vi "DriveNetwork.vi"(8 "error in (no error)":errorcluster) -> (0 "error out":errorcluster)   [LabVIEW 2023]
doc: "Network for Drive\n\nInputs:\n -- Error in -- Error cluster -- propagated error input\n\nOutputs:\n -- Error out -- Error cluster -- progated error output"
uses:
  DriveGlobal.vi
  <vilib>/Rock Robotics/Network Tables/NT Get Topic.vi
  <vilib>/Rock Robotics/Network Tables/NT Get PublishHandle.vi
  <vilib>/Rock Robotics/Network Tables/NT_LL_Write Number.vi
  <vilib>/Rock Robotics/Network Tables/NT Check Errors.vi
  <vilib>/Rock Robotics/WPI/ThirdParty/JAS_Junk/TrajLib/Trajectory_Library.lvlib
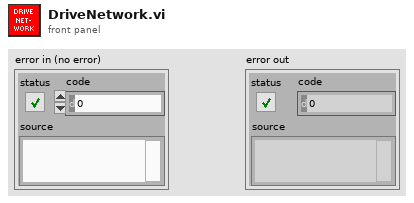
[diagram p1: front panel]
types:
  T1 = typedef "Trajectory_Library.lvlib/SWERVE_DRIVE_KINEMATICS.ctl" = cluster{"NumModules":i32, "InverseKinematics":T2, "ForwardKinematics":T2, "Modules":T3[], "PrevCoR":T3, "SavedModuleStates":T4[]}
  T2 = typedef "NI_Matrix.lvlib/RealMatrix.ctl" = dbl[][]
  T3 = typedef "Trajectory_Library.lvlib/TRANSLATION2D.ctl" = cluster{"X":dbl, "Y":dbl}
  T4 = typedef "Trajectory_Library.lvlib/SWERVE_DRIVE_MODULE_STATE.ctl" = cluster{"Speed":dbl, "Angle":T5}
  T5 = typedef "Trajectory_Library.lvlib/ROTATION2D.ctl" = cluster{"VALUE":dbl, "COS":dbl, "SIN":dbl}
  T6 = typedef "Trajectory_Library.lvlib/CHASSIS_SPEEDS.ctl" = cluster{"vX":dbl, "vY":dbl, "vOmega":dbl}
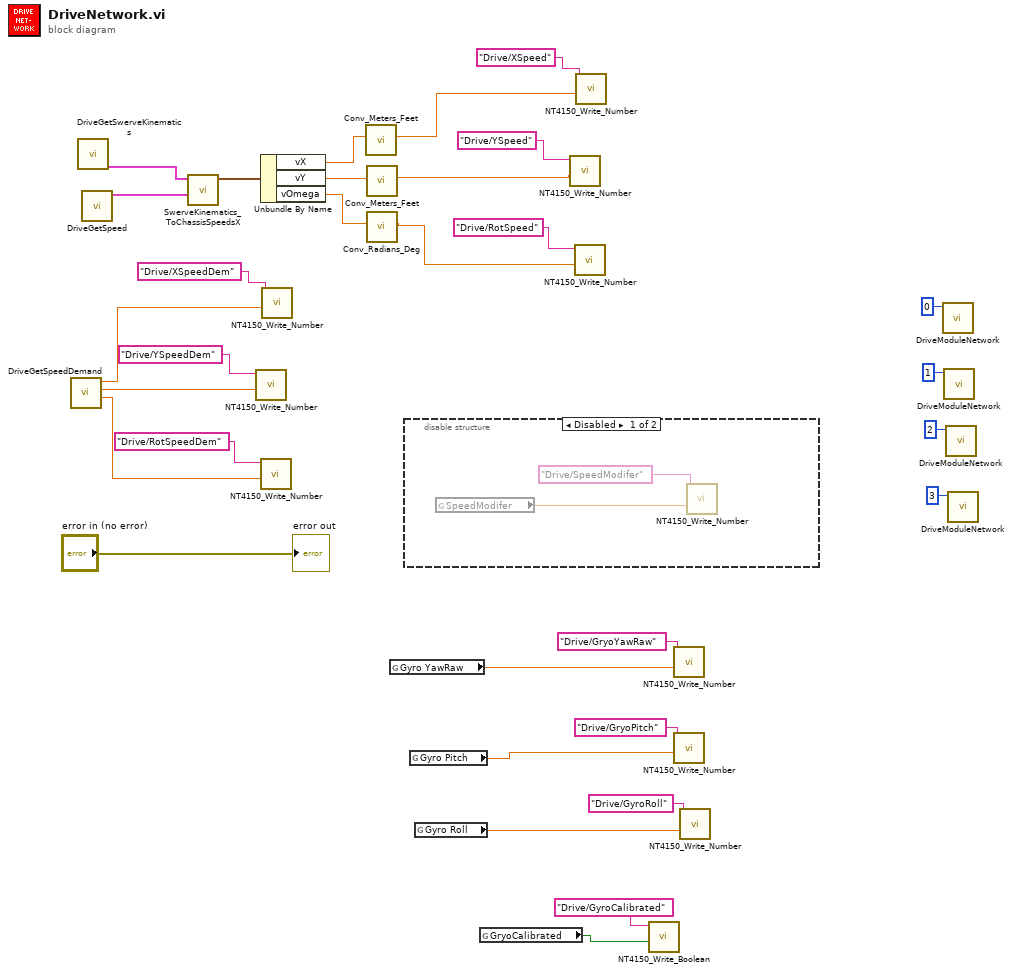
[diagram p0: block diagram]
diagram:
  n1 = call "DriveGetSpeedDemand.vi"() -> ("vOmega"=w17:dbl, "vY"=w29:dbl, "vX"=w30:dbl)  [unwired: 8 in, 1 out]
  n2 = call "DriveGetSwerveKinematics.vi"() -> ("SWERVE_DRIVE_KINEMATICS"=w12:T1)  [unwired: 11 in]
  n3 = call "DriveGetSpeed.vi"() -> ("Swerve__Drive_Modual_States"=w11:T4[])  [unwired: 11 in]
  n4 = call <vilib>:"SwerveKinematics_ToChassisSpeedsX.vi"("WheelStates"=w11, "in SWERVE_DRIVE_KINEMATICS"=w12) -> ("Chassis Speed"=w10:T6)  [unwired: 9 in]
  n5 = call "NT4150_Write_Number.vi"("value"=w29, "name"="Drive/YSpeedDem") -> ()  [unwired: 9 in, 1 out]
  n6 = Unbundle By Name(w10) -> ("vX"=w9:dbl, "vY"=w8:dbl, "vOmega"=w7:dbl)
  n7 = call "NT4150_Write_Number.vi"("value"=w17, "name"="Drive/RotSpeedDem") -> ()  [unwired: 9 in, 1 out]
  n8 = call "NT4150_Write_Number.vi"("value"=w30, "name"="Drive/XSpeedDem") -> ()  [unwired: 9 in, 1 out]
  n9 = call <vilib>:"Conv_Meters_Feet.vi"("Meters"=w9) -> ("Feet"=w1:dbl)  [unwired: 10 in]
  n10 = call <vilib>:"Conv_Meters_Feet.vi"("Meters"=w8) -> ("Feet"=w2:dbl)  [unwired: 10 in]
  n11 = call <vilib>:"Conv_Radians_Deg.vi"("Radians"=w7) -> ("Degrees"=w3:dbl)  [unwired: 10 in]
  n12 = global read "DriveGlobal.vi" "Gyro YawRaw"() -> (w23:dbl)
  n13 = disable-structure shown="Disabled" {
    frame Disabled {
      n14 = global read "DriveGlobal.vi" "SpeedModifer"() -> (w32:dbl)
      n15 = call "NT4150_Write_Number.vi"("value"=w32, "name"="Drive/SpeedModifer") -> ()  [unwired: 9 in, 1 out]
    }
    frame Enabled {
    }
  }
  n16 = global read "DriveGlobal.vi" "Gyro Pitch"() -> (w24:dbl)
  n17 = global read "DriveGlobal.vi" "Gyro Roll"() -> (w25:dbl)
  n18 = global read "DriveGlobal.vi" "GryoCalibrated"() -> (w19:bool)
  n19 = call "NT4150_Write_Number.vi"("value"=w2, "name"="Drive/YSpeed") -> ()  [unwired: 9 in, 1 out]
  n20 = call "NT4150_Write_Number.vi"("value"=w3, "name"="Drive/RotSpeed") -> ()  [unwired: 9 in, 1 out]
  n21 = call "NT4150_Write_Number.vi"("value"=w1, "name"="Drive/XSpeed") -> ()  [unwired: 9 in, 1 out]
  n22 = call "NT4150_Write_Boolean.vi"("value"=w19, "name"="Drive/GyroCalibrated") -> ()  [unwired: 9 in, 1 out]
  n23 = call "NT4150_Write_Number.vi"("value"=w23, "name"="Drive/GryoYawRaw") -> ()  [unwired: 9 in, 1 out]
  n24 = call "NT4150_Write_Number.vi"("value"=w24, "name"="Drive/GryoPitch") -> ()  [unwired: 9 in, 1 out]
  n25 = call "NT4150_Write_Number.vi"("value"=w25, "name"="Drive/GyroRoll") -> ()  [unwired: 9 in, 1 out]
  n26 = call "DriveModuleNetwork.vi"("Module"=0) -> ()  [unwired: 10 in, 1 out]
  n27 = call "DriveModuleNetwork.vi"("Module"=1) -> ()  [unwired: 10 in, 1 out]
  n28 = call "DriveModuleNetwork.vi"("Module"=2) -> ()  [unwired: 10 in, 1 out]
  n29 = call "DriveModuleNetwork.vi"("Module"=3) -> ()  [unwired: 10 in, 1 out]
  "error out" <- "error in (no error)"
